vi "NanotecSMCPDDriver.errorQuery.vi"(0 "VISA resource name":refnum<visa-resource-name>, 1 "contollerID":i32=-1, 5 "error in (no error)":errorcluster) -> (14 "VISA resource name out":refnum<visa-resource-name>, 15 "contollerID out":i32=-1, 16 "Error Code":i32[](array[numeric]), 17 "Error Message":string, 19 "error out":errorcluster)   [LabVIEW 2014, in "NanotecSMCPDDriver.lvlib"]
doc: "Queries the instrument for any errors in the instrument's error queue. It will continue to read errors until all errors have been read from the instrument. Any errors will be returned in the <B>error out</B> control.\n\nNote:\nThis VI is called automatically by most driver VIs so it is not usually necessary to call this in an application."
uses:
  NanotecSMCPDDriver.lvlib
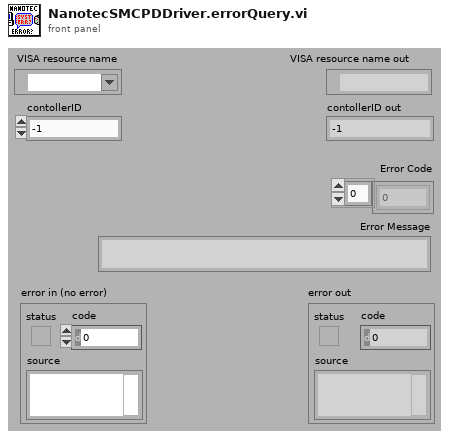
[diagram p1: front panel]
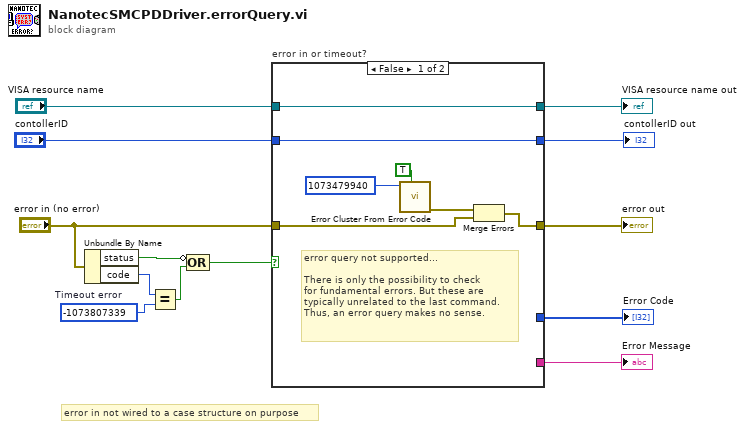
[diagram p0: block diagram]
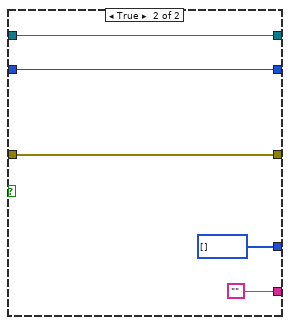
[diagram p2: hidden frame]
diagram:
  w8 = -1073807339  # Timeout error
  # "error in not wired to a case structure on purpose"
  n1 = Unbundle By Name("error in (no error)") -> ("status"=w9:bool, "code"=w6:i32)
  n2 = Equal?(x=w6, y=w8) -> (x = y?=w7:bool)
  n3 = Compound Arithmetic op=OR(invert w9, w7) -> (w5:bool)
  n4 = case "error in or timeout?" shown="False" w5 {
    tunnel: [w17 w25] -> w13
    tunnel: "VISA resource name" -> [w17 w25]
    tunnel: "error in (no error)" -> [w18 w24]
    tunnel: [w20 w24] -> w11
    tunnel: [_ "" ("Empty String Constant")] -> w4
    tunnel: [_ i32[] []] -> w3
    tunnel: "contollerID" -> [w16 w21]
    tunnel: [w16 w21] -> w1
    frame False {
      # "error query not supported...\n\nThere is only the possibility to check\nfor fundamental errors. But these are\ntypically unrelated to the last command.\nThus, an error query makes no sense."
      n5 = call <vilib>:"Error Cluster From Error Code.vi"("show call chain? (False)"=TRUE, "error code (0)"=1073479940 ("Code")) -> ("error out"=w19:errorcluster)  [unwired: 7 in]
      n6 = Merge Errors(w19, w18) -> (w20:errorcluster)
    }
    frame True {
    }
  }
  "VISA resource name out" <- w13
  "error out" <- w11
  "Error Message" <- w4
  "Error Code" <- w3
  "contollerID out" <- w1
